vi "ADQ214 Memory Dump.vi"(0 "adq_cu_ptr":u32, 1 "buffer":string, 5 "adq214_num":i32, 7 "StartAddress":u32, 9 "EndAddress":u32, 11 "error in (no error)":errorcluster, 12 "bufctr":u32) -> (3 "buffer out":string, 4 "adq_cu_ptr out":u32, 6 "function return":u32, 14 "bufctr out":u32, 15 "error out":errorcluster)   [LabVIEW 8.6, in "ADQAPI.lvlib"]
doc: "extern \"C\" __declspec(dllimport) unsigned int ADQ214_MemoryDump(void* adq_cu_ptr, int adq214_num, unsigned int StartAddress, unsigned int EndAddress, unsigned char* buffer, unsigned int *bufctr);"
uses:
  F/HRT/Sp Devices Thesis/ADQ-214 project (H R)/ADQAPI.lvlib
  F:/HRT/Sp Devices Thesis/ADQ-214 project (H R)/ADQAPI.dll
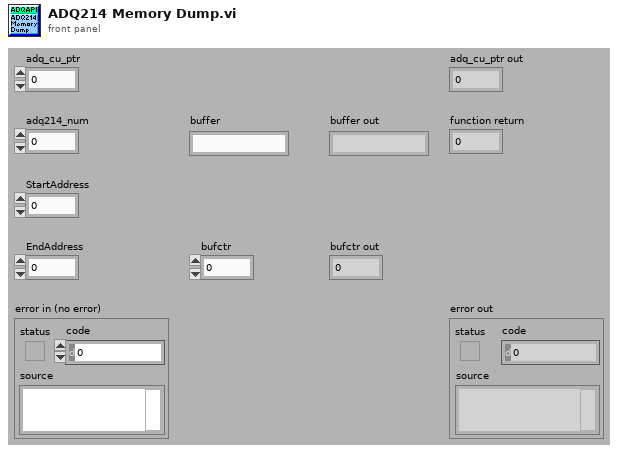
[diagram p1: front panel]
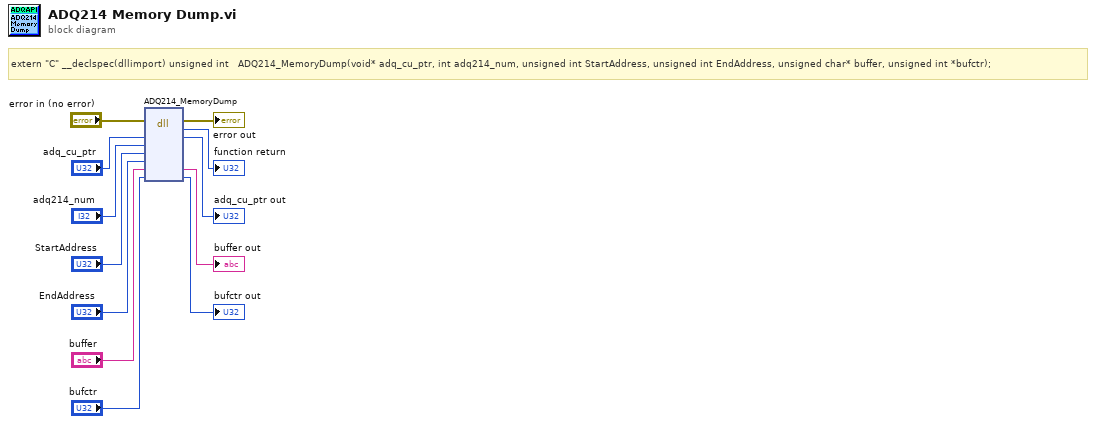
[diagram p0: block diagram]
diagram:
  # "extern \"C\" __declspec(dllimport) unsigned int   ADQ214_MemoryDump(void* adq_cu_ptr, int adq214_num,\tunsigned int StartAddress, unsigned int EndAddress, unsigned char* buffer, unsigned int *bufctr);"
  n1 = dll-call lib="F:/HRT/Sp Devices Thesis/ADQ-214 project (H R)/ADQAPI.*" fn="ADQ214_MemoryDump"(error in="error in (no error)", "adq_cu_ptr"="adq_cu_ptr", "adq214_num"="adq214_num", "StartAddress"="StartAddress", "EndAddress"="EndAddress", "buffer"="buffer", "bufctr"="bufctr") -> (error out=→"error out":errorcluster, →"function return":u32, "adq_cu_ptr"=→"adq_cu_ptr out":u32, "buffer"=→"buffer out":string, "bufctr"=→"bufctr out":u32)  [unwired: 5 in, 1 out]
